vi "Network Sink - Module 1.vi"() -> ()   [LabVIEW 2017, in "Network Logger Examples.lvlib"]
uses:
  <vilib>/gpm_packages/@cs/event-logger/Examples/Examples/Network Logger Examples.lvlib
  <vilib>/gpm_packages/@cs/event-logger/Source/Composed Log/Types/Log Level.ctl
  <vilib>/gpm_packages/@cs/event-logger/Source/Composed Log/LoggerReference/LoggerReference.lvclass/LoggerReference.ctl
  b558ab63-4aa2-4cbd-b208-fa7bab295c73.vi
  <vilib>/gpm_packages/@cs/event-logger/Source/Composed Log/LoggerReference/Return Aggregate Queues.vi
  <vilib>/gpm_packages/@cs/event-logger/Source/Composed Log/LoggerReference/Add Aggregate Log.vi
  b558ab63-4aa2-4cbd-b208-fa7bab295c73.vi/885c6045-dbe6-450b-aeed-5b35f96d23a7.vi
  <vilib>/gpm_packages/@cs/event-logger/Source/Composed Log/LoggerReference/Log.vi
  <vilib>/gpm_packages/@cs/event-logger/Source/Composed Log/LoggerReference/Get Valid Event Time.vi
  <vilib>/gpm_packages/@cs/event-logger/Source/Composed Log/LoggerReference/Send Add Sink.vi
  <vilib>/gpm_packages/@cs/event-logger/Source/Composed Log/LoggerReference/Remove Stale Logs.vi
  <vilib>/gpm_packages/@cs/event-logger/Source/String Control Sink/String Control Sink.lvclass
  C:/Program Files/National Instruments/LabVIEW 2017/vi.lib/gpm_packages/@cs/event-logger/Source/Composed Log/Log Sink/Log Sink.lvclass
  <vilib>/gpm_packages/@cs/event-logger/Source/Network Sink/Network Sink/Network Sink.lvclass
  <vilib>/gpm_packages/@cs/event-logger/Source/Composed Log/Application Logger/Launch Worker Loop.vi
  <vilib>/gpm_packages/@cs/event-logger/Source/Composed Log/LoggerReference/Initialize Logger Instance.vi
  <vilib>/gpm_packages/@cs/event-logger/Source/Composed Log/LoggerReference/LoggerReference.lvclass
  <vilib>/gpm_packages/@cs/event-logger/Source/Composed Log/IErrorFormat/IErrorFormat.lvclass
  <vilib>/gpm_packages/@cs/event-logger/Source/Composed Log/Log Sink/Log Sink.lvclass
  <vilib>/gpm_packages/@cs/event-logger/Source/Composed Log/Composed Log.lvlib
panel:
  in  "Event Level":T1(ring)
  in  "Data To Log":string
  in  "Source":string="User"
  in  "Log":bool
  in  "Local Event Log":string
  # "Run the VI. If it isn't already running, start the VI - Network Sink - Log Aggregator. Use the log custom event to add user defined log messages. Observe that the log aggregator catches events from this module."
  # "Log Custom Event"
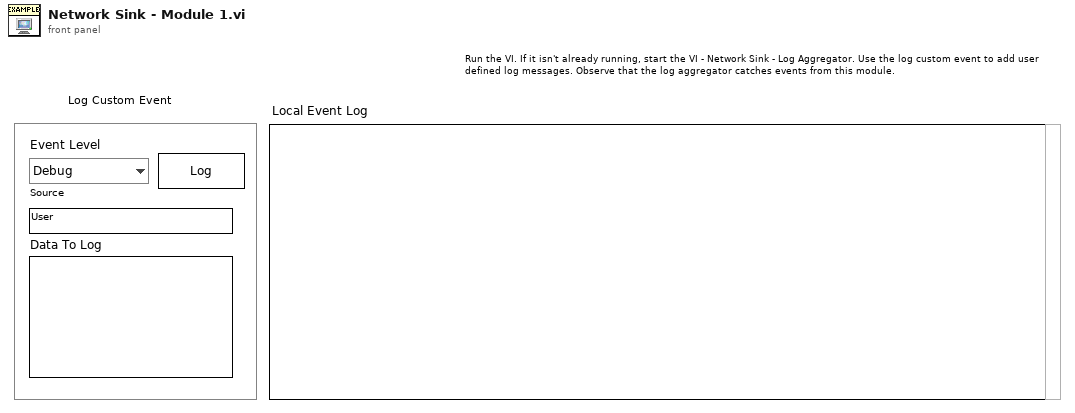
[diagram p1: front panel]
types:
  T1 = enum16{"Debug", "Info", "Warning", "Error", "Critical"}
  T2 = typedef "Composed Log.lvlib/Log Level.ctl" = enum16{"Debug", "Info", "Warning", "Error", "Critical"}
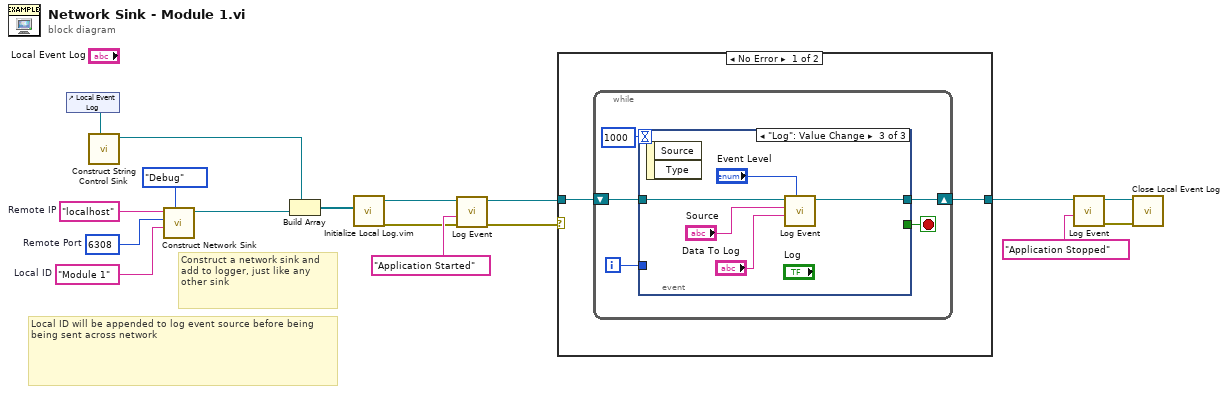
[diagram p0: block diagram]
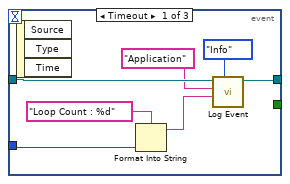
[diagram p2: hidden frame]
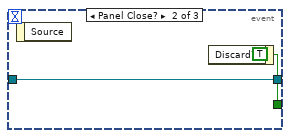
[diagram p3: hidden frame]
diagram:
  w12 = u16 6308  # Remote Port
  w13 = "Module 1"  # Local ID
  w14 = "localhost"  # Remote IP
  # "Construct a network sink and add to logger, just like any other sink"
  # "Local ID will be appended to log event source before being being sent across network"
  n1 = control-ref of="Local Event Log"() -> (w16:refnum<vi>)
  n2 = call <vilib>:"Construct String Control Sink.vi"("Str Refnum"=w16) -> ("String Control Sink out"=w17:refnum<class "String Control Sink.lvclass">)  [unwired: 10 in]
  n3 = call <vilib>:"Construct Network Sink.vi"("LogLevel"=Log_Level."Debug", "Local ID"=w13, "Remote Port"=w12, "Remote IP"=w14) -> ("Network Sink out"=w8:refnum<class "Network Sink.lvclass">)  [unwired: 7 in]
  n4 = Build Array(w17, w8) -> (w15:refnum<class "Log Sink.lvclass">[])
  n5 = call "Initialize Local Log.vim"("Startup Sink(s)"=w15) -> ("error out"=w3:errorcluster, "Log Instance Reference"=w6:refnum<class "LoggerReference.lvclass">)  [unwired: 8 in, 1 out]
  n6 = call <vilib>:"Log Event.vi"("error in (no error)"=w3, "Data To Log"="Application Started", "Log Instance"=w6) -> ("error out"=w4:errorcluster, "Log Instance Out"=w5:refnum<class "LoggerReference.lvclass">)  [unwired: 7 in]
  n7 = case shown="No Error" w4 {
    tunnel: w5 -> [w19 w39]
    tunnel: [w18 w39] -> w11
    frame No Error {
      n8 = while {
        shift-right: [w22] -> w18
        shift-left: w19 -> [w23]
        i -> [w20]
        stop <- w24 stop-if-true
        n9 = event shown="[2] \"Log\": Value Change" {
          selector: _ -> [_ _ _]
          dyn-events: _ -> [_ _ _]
          timeout: 1000 -> [_ _ _]
          tunnel: [_ w33 _] -> w24
          tunnel: w23 -> [w31 w32 w38]
          tunnel: [w29 w32 w36] -> w22
          tunnel: w20 -> [w27 _ _]
          event Timeout {
            n10 = event-data() -> ()  [unwired: 1 in, 3 out]
            n11 = Format Into String(format string="Loop Count : %d" ("Data To Log"), w27) -> (resulting string=w25:string)  [unwired: 2 in, 1 out]
            n12 = call <vilib>:"Log Event.vi"("Event Level"=Log_Level."Info", "Data To Log"=w25, "SourceID"="Application", "Log Instance"=w31) -> ("Log Instance Out"=w29:refnum<class "LoggerReference.lvclass">)  [unwired: 6 in, 1 out]
          }
          event Panel Close? {
            w33 = TRUE ("Discard?")
            n13 = event-data() -> ()  [unwired: 1 in, 1 out]
            n14 = event-data("Discard?"=w33) -> ()  [unwired: 1 in, 1 out]
          }
          event "Log": Value Change {
            n15 = event-data() -> ()  [unwired: 1 in, 2 out]
            n16 = call <vilib>:"Log Event.vi"("Event Level"="Event Level", "Data To Log"="Data To Log", "SourceID"="Source", "Log Instance"=w38) -> ("Log Instance Out"=w36:refnum<class "LoggerReference.lvclass">)  [unwired: 6 in, 1 out]
          }
        }
      }
    }
    frame Error {
    }
  }
  n17 = call <vilib>:"Log Event.vi"("Data To Log"="Application Stopped", "Log Instance"=w11) -> ("error out"=w2:errorcluster, "Log Instance Out"=w10:refnum<class "LoggerReference.lvclass">)  [unwired: 8 in]
  n18 = call <vilib>:"Close Local Event Log.vi"("error in (no error)"=w2, "Log Instance"=w10) -> ()  [unwired: 9 in, 1 out]
